vi "Part 1.vi"(11 "Input":string) -> (3 "Output":i64)   [LabVIEW 2021]
uses:
  3f712b8c-fb5b-4fbc-874d-0abea8c1e874.vi
  <userlib>/_OpenG.lib/string/string.llb/Convert EOLs (String)__ogtk.vi
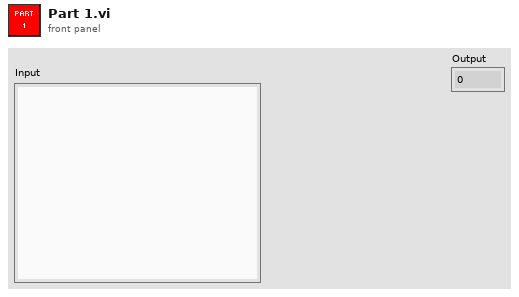
[diagram p1: front panel]
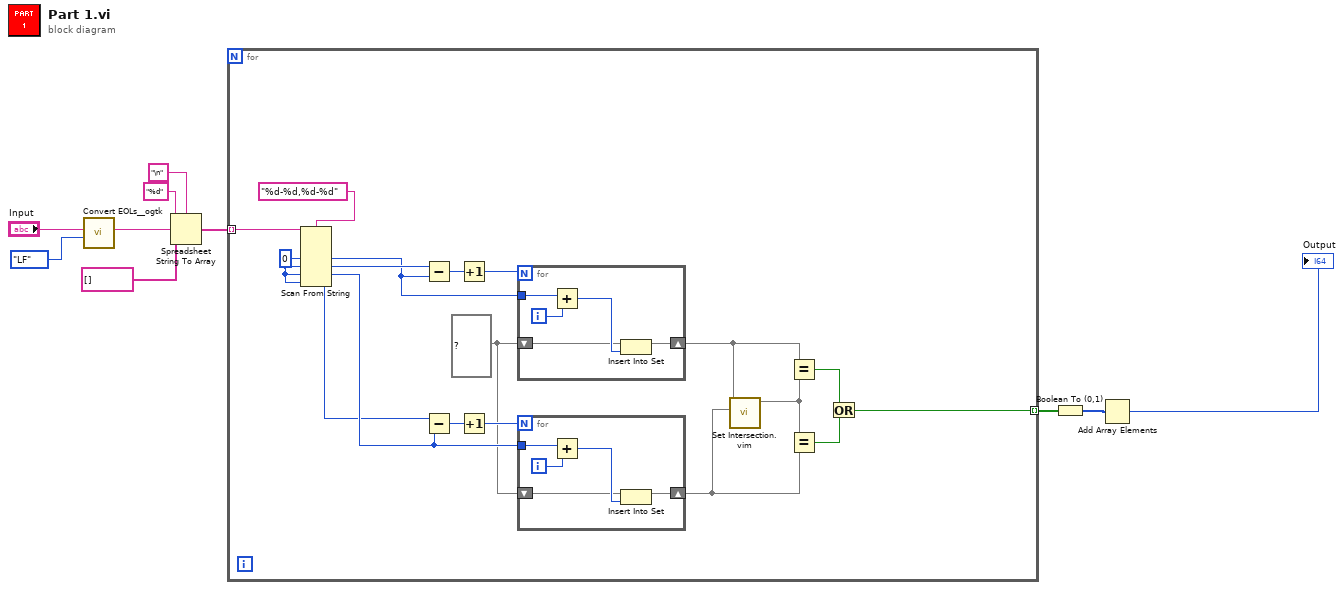
[diagram p0: block diagram]
diagram:
  n1 = call-poly <userlib>:"Convert EOLs__ogtk.vi"("Convert to:"=enum16{"CR", "LF", "CRLF"}."LF", "String in"="Input") -> ("String out"=w6:string)  [unwired: 9 in]
  n2 = Spreadsheet String To Array(delimiter (Tab)="\n", format string="%d", spreadsheet string=w6, array type (2D Dbl)=string[] []) -> (array=w4:string[])
  n3 = for {
    tunnel: w4 -> [w28] mode=indexing
    tunnel: [w11] -> w3 mode=indexing
    w17 = set{i64} {} ("set out")
    w26 = i64 0 ("default value 1")
    n4 = Scan From String(format string="%d-%d,%d-%d", input string=w28, default 1=w26, default 2=w26, default 3=w26, default 4=w26) -> (output 1=w22:i64, output 2=w25:i64, output 3=w20:i64, output 4=w19:i64)  [unwired: 2 in, 3 out]
    n5 = Subtract(x=w25, y=w22) -> (x-y=w24:i64)
    n6 = Subtract(x=w19, y=w20) -> (x-y=w21:i64)
    n7 = Increment(x=w24) -> (x+1=w23:i64)
    n8 = Increment(x=w21) -> (x+1=w18:i64)
    n9 = for {
      N: w23 -> [_]
      tunnel: w22 -> [w38]
      shift-right: [w34] -> w16
      shift-left: w17 -> [w35]
      i -> [w37]
      n10 = Add(x=w38, y=w37) -> (x+y=w36:i64)
      n11 = Insert Into Set(10:w36, 11:w35) -> (3:w34:set{i64})  [unwired: 1 out]
    }
    n12 = for {
      N: w18 -> [_]
      tunnel: w20 -> [w33]
      shift-right: [w29] -> w14
      shift-left: w17 -> [w30]
      i -> [w32]
      n13 = Add(x=w33, y=w32) -> (x+y=w31:i64)
      n14 = Insert Into Set(10:w31, 11:w30) -> (3:w29:set{i64})  [unwired: 1 out]
    }
    n15 = call "Set Intersection.vim"("set 2"=w14, "set 1"=w16) -> ("intersection"=w15:set{i64})  [unwired: 9 in]
    n16 = Equal?(x=w16, y=w15) -> (x = y?=w13:bool)
    n17 = Equal?(x=w15, y=w14) -> (x = y?=w12:bool)
    n18 = Or(x=w13, y=w12) -> (x .or. y?=w11:bool)
  }
  n19 = Boolean To (0,1)(Boolean=w3) -> (0, 1=w2:i16[])
  n20 = Add Array Elements(numeric array=w2) -> (sum=→"Output":i16)
